vi "InvFilter-Check Parameters.vi"(0 "InvFilt Params":T1) -> (15 "error out":errorcluster)   [LabVIEW 2020]
uses:
  InvFilt-Params.ctl
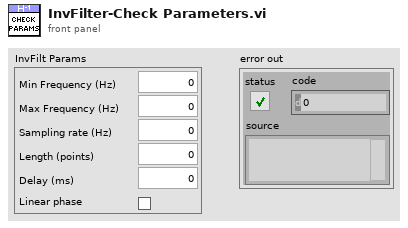
[diagram p1: front panel]
types:
  T1 = typedef "InvFilt-Params.ctl" = cluster{"Min Frequency (Hz)":dbl, "Max Frequency (Hz)":dbl, "Length (points)":i32, "Sampling rate (Hz)":dbl, "Delay (ms)":dbl, "Linear phase":bool}
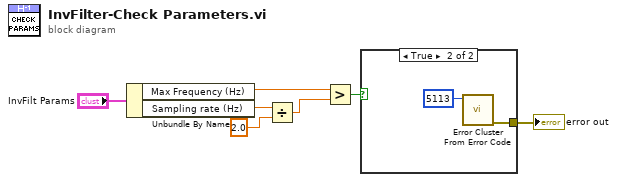
[diagram p0: block diagram]
diagram:
  n1 = Unbundle By Name("InvFilt Params") -> ("Max Frequency (Hz)"=w6:dbl, "Sampling rate (Hz)"=w5:dbl)
  n2 = Divide(x=w5, y=2.0) -> (x/y=w3:dbl)
  n3 = Greater?(x=w6, y=w3) -> (0:w2:bool)
  n4 = case shown="True" w2 {
    tunnel: [_ w9] -> w1
    frame False {
    }
    frame True {
      n5 = call <vilib>:"Error Cluster From Error Code.vi"("error code (0)"=5113) -> ("error out"=w9:errorcluster)  [unwired: 8 in]
    }
  }
  "error out" <- w1
